vi "Log Output.vi"(6 "VI Name":string, 7 "error in (no error)":errorcluster caption="エラー入力 (エラーなし)" {"code" format="%.0x"}, 10 "Result Log Reference":refnum<vi>) -> (0 "error out":errorcluster caption="エラー出力" {"code" format="%.0x"}, 3 "Result Log Reference Out":refnum<vi>)   [LabVIEW 2020]
panel:
  out "Appending Strings(debug)":string
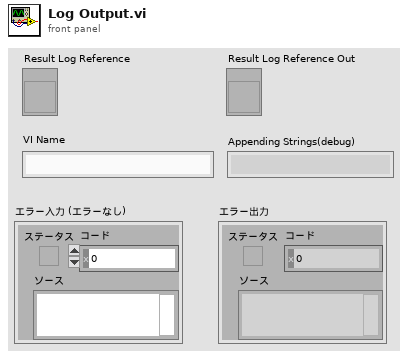
[diagram p1: front panel]
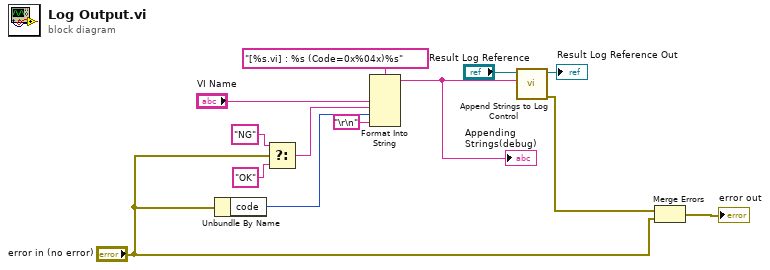
[diagram p0: block diagram]
diagram:
  n1 = Unbundle By Name("error in (no error)") -> ("code"=w8:i32)
  n2 = Select(t="NG" ("Œ`Ž®•¶Žš—ñ"), s="error in (no error)", f="OK" ("Œ`Ž®•¶Žš—ñ")) -> (s? t:f=w9:string)
  n3 = Format Into String(format string="[%s.vi] : %s (Code=0x%04x)%s" ("Œ`Ž®•¶Žš—ñ"), "VI Name", w9, w8, "\r\n") -> (resulting string=w6:string)  [unwired: 2 in, 1 out]
  "Appending Strings(debug)" <- w6
  n4 = call "Append Strings to Log Control.vi"("Appending Strings"=w6, "Result Log Reference"="Result Log Reference") -> ("エラー出力"=w4:errorcluster, "Result Log Reference Out"=→"Result Log Reference Out":refnum<vi>)  [unwired: 8 in]
  n5 = Merge Errors(w4, "error in (no error)") -> (→"error out":errorcluster)
